vi "Read Topic Info.vi"(11 "Topic in":refnum<class "Topic.lvclass">) -> (0 "Last Publication Time":timestamp, 1 "Enqueuer (UID)":refnum<class "Message Enqueuer.lvclass">, 2 "Name":string, 3 "Type":string)   [LabVIEW 2017, in "Mediator.lvlib" / "Topic.lvclass"]
doc: "<License>\nCopyright © 2017 Composed Systems, LLC | All rights reserved\nwww.composed.io\n\nAuthor: Ethan Stern <ethan.stern@composed.io>\n\nThis software is provided \"AS IS\" WITHOUT WARRANTIES, either express or implied, AND IS FOR EDUCATIONAL PURPOSES ONLY.\n</License>"
uses:
  Topic.lvclass
  C:/Program Files (x86)/National Instruments/LabVIEW 2017/vi.lib/ActorFramework/Actor/Actor.lvclass
  <vilib>/ActorFramework/Message Enqueuer/Message Enqueuer.lvclass
  <vilib>/ActorFramework/Actor/Actor.lvclass/Actor.ctl
  <vilib>/ActorFramework/Message Enqueuer/Message Enqueuer.lvclass/Message Enqueuer.ctl
  Topic.lvclass/Topic.ctl
  <vilib>/ActorFramework/Message Enqueuer/Init from Existing Queue.vi
  <vilib>/ActorFramework/Actor/Actor.lvclass
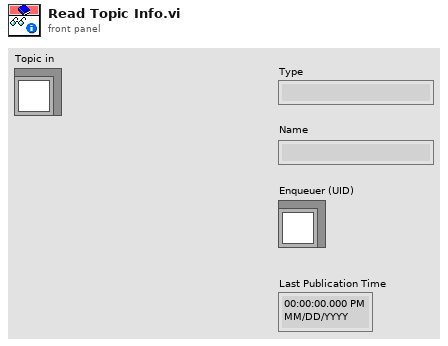
[diagram p1: front panel]
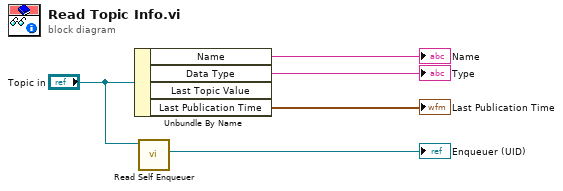
[diagram p0: block diagram]
diagram:
  n1 = Unbundle By Name("Topic in") -> ("Name"=→"Name":string, "Data Type"=→"Type":string, "Last Publication Time"=→"Last Publication Time":timestamp)  [unwired: 1 out]
  n2 = call <vilib>:"Read Self Enqueuer.vi"("Actor"="Topic in") -> ("Self Enqueuer"=→"Enqueuer (UID)":refnum<class "Message Enqueuer.lvclass">)  [unwired: 10 in]
